vi "Matrix Inverse.vi"(2 "n":i32, 3 "A":sgl[](array[numeric])) -> (0 "divide by zero detected":bool, 1 "inv(A)":sgl[](array[numeric]))   [LabVIEW 2020]
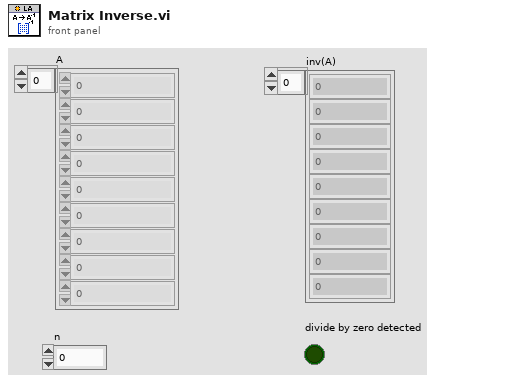
[diagram p1: front panel]
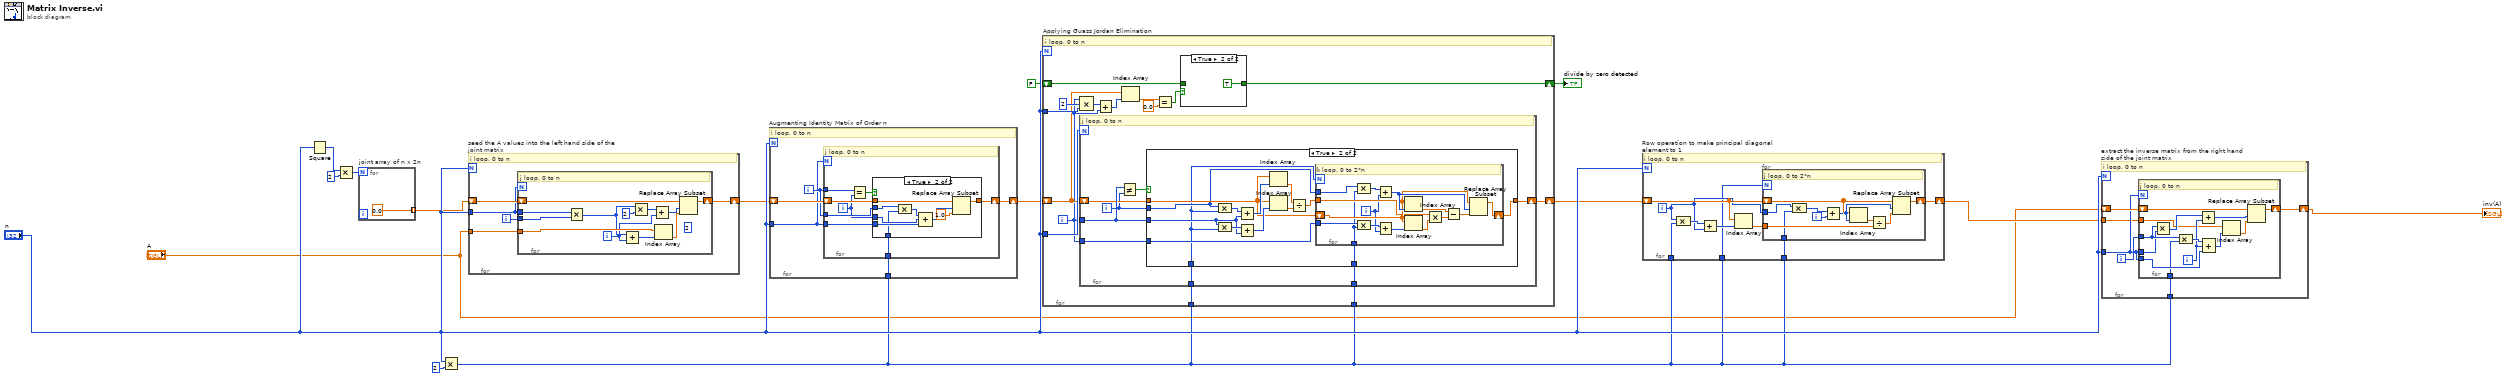
[diagram p0: block diagram]
diagram:
  n1 = Square(x="n") -> (x^2=w14:i32)
  n2 = Multiply(x=w14, y=2) -> (x*y=w2:i32)
  n3 = for "joint array of n x 2n" {
    N: w2 -> [_]
    tunnel: [sgl 0.0] -> w3 mode=indexing
  }
  n4 = Multiply(x="n", y=2) -> (x*y=w13:i32)
  n5 = for "seed the A values into the left hand side of the joint matrix" {
    N: "n" -> [_]
    shift-right: [w20] -> w4
    shift-left: w3 -> [w21]
    tunnel: "n" -> [w19]
    tunnel: "A" -> [w18]
    i -> [w17]
    # "i loop, 0 to n"
    n6 = for {
      N: w19 -> [_]
      shift-right: [w32] -> w20
      shift-left: w21 -> [w33]
      tunnel: w19 -> [w29]
      tunnel: w18 -> [w31]
      tunnel: w17 -> [w30]
      i -> [w23]
      (unwired) 2
      # "j loop, 0 to n"
      n7 = Multiply(x=w29, y=w30) -> (x*y=w25:i32)
      n8 = Add(x=w25, y=w23) -> (x+y=w28:i32)
      n9 = Multiply(x=w25, y=2) -> (x*y=w24:i32)
      n10 = Add(x=w24, y=w23) -> (x+y=w22:i32)
      n11 = Index Array(array=w31, index=w28) -> (element=w27:sgl)
      n12 = Replace Array Subset(array=w33, new element=w27, index=w22) -> (w32:sgl[])
    }
  }
  n13 = for "Augmenting Identity Matrix of Order n" {
    N: "n" -> [_]
    shift-right: [w37] -> w7
    shift-left: w4 -> [w38]
    tunnel: "n" -> [w35]
    tunnel: w13 -> [w34]
    i -> [w36]
    # "i loop, 0 to n"
    n14 = for {
      N: w35 -> [_]
      tunnel: w36 -> [w46]
      shift-right: [w43] -> w37
      shift-left: w38 -> [w44]
      tunnel: w36 -> [w42]
      tunnel: w35 -> [w41]
      tunnel: w34 -> [w39]
      i -> [w40]
      # "j loop, 0 to n"
      n15 = Equal?(x=w46, y=w40) -> (x = y?=w45:bool)
      n16 = case shown="True" w45 {
        tunnel: w44 -> [w47 w56]
        tunnel: [w47 w53] -> w43
        tunnel: w42 -> [_ w54]
        tunnel: w41 -> [_ w50]
        tunnel: w40 -> [_ w51]
        tunnel: w39 -> [_ w48]
        frame False {
        }
        frame True {
          n17 = Compound Arithmetic op=MULTIPLY(w54, w48) -> (w52:i32)
          n18 = Compound Arithmetic op=ADD(w52, w51, w50) -> (w49:i32)
          n19 = Replace Array Subset(array=w56, new element=sgl 1.0 ("new element/subarray"), index=w49) -> (w53:sgl[])
        }
      }
    }
  }
  n20 = for "Applying Guass Jordan Elimination" {
    N: "n" -> [_]
    tunnel: "n" -> [w69]
    shift-right: [w63] -> w6
    shift-left: FALSE -> [w64]
    tunnel: "n" -> [w62]
    shift-right: [w59] -> w8
    shift-left: w7 -> [w61]
    tunnel: w13 -> [w58]
    tunnel: w13 -> [w57]
    i -> [w60]
    # "i loop, 0 to n"
    n21 = Compound Arithmetic op=MULTIPLY(w60, 2 ("value"), w69) -> (w68:i32)
    n22 = for {
      N: w62 -> [_]
      tunnel: w60 -> [w79]
      tunnel: w60 -> [w75]
      shift-right: [w74] -> w59
      shift-left: w61 -> [w78]
      tunnel: w58 -> [w73]
      tunnel: w57 -> [w72]
      i -> [w76]
      # "j loop, 0 to n"
      n23 = Not Equal?(x=w79, y=w76) -> (x != y?=w77:bool)
      n24 = case shown="True" w77 {
        tunnel: w79 -> [_ w88]
        tunnel: w78 -> [w80 w87]
        tunnel: w76 -> [_ w86]
        tunnel: w75 -> [_ w84]
        tunnel: [w80 w83] -> w74
        tunnel: w73 -> [_ w82]
        tunnel: w72 -> [_ w81]
        frame False {
        }
        frame True {
          n25 = Compound Arithmetic op=MULTIPLY(w86, w82) -> (w94:i32)
          n26 = Compound Arithmetic op=MULTIPLY(w88, w82) -> (w90:i32)
          n27 = Add(x=w94, y=w88) -> (x+y=w93:i32)
          n28 = Add(x=w90, y=w88) -> (x+y=w89:i32)
          n29 = Index Array(array=w87, index=w93) -> (element=w92:sgl)
          n30 = Index Array(array=w87, index=w89) -> (element=w91:sgl)
          n31 = Divide(x=w92, y=w91) -> (x/y=w85:sgl)
          n32 = for {
            N: w82 -> [_]
            tunnel: w86 -> [w108]
            tunnel: w85 -> [w104]
            tunnel: w84 -> [w101]
            shift-right: [w96] -> w83
            shift-left: w87 -> [w106]
            tunnel: w81 -> [w95]
            i -> [w102]
            # "k loop, 0 to 2*n"
            n33 = Compound Arithmetic op=MULTIPLY(w108, w95) -> (w109:i32)
            n34 = Compound Arithmetic op=MULTIPLY(w101, w95) -> (w103:i32)
            n35 = Add(x=w109, y=w102) -> (x+y=w107:i32)
            n36 = Add(x=w103, y=w102) -> (x+y=w100:i32)
            n37 = Index Array(array=w106, index=w107) -> (element=w98:sgl)
            n38 = Index Array(array=w106, index=w100) -> (element=w105:sgl)
            n39 = Multiply(x=w104, y=w105) -> (x*y=w99:sgl)
            n40 = Subtract(x=w98, y=w99) -> (x-y=w97:sgl)
            n41 = Replace Array Subset(array=w106, new element=w97, index=w107) -> (w96:sgl[])
          }
        }
      }
    }
    n42 = Add(x=w68, y=w60) -> (x+y=w67:i32)
    n43 = Index Array(array=w61, index=w67) -> (element=w66:sgl)
    n44 = Equal?(x=w66, y=sgl 0.0) -> (x = y?=w65:bool)
    n45 = case shown="True" w65 {
      tunnel: w64 -> [w110 _]
      tunnel: [w110 TRUE] -> w63
      frame False {
      }
      frame True {
      }
    }
  }
  "divide by zero detected" <- w6
  n46 = for "Row operation to make principal diagonal element to 1" {
    N: "n" -> [_]
    shift-right: [w115] -> w11
    shift-left: w8 -> [w118]
    tunnel: w13 -> [w114]
    tunnel: w13 -> [w113]
    tunnel: w13 -> [w112]
    i -> [w117]
    # "i loop, 0 to n"
    n47 = Compound Arithmetic op=MULTIPLY(w117, w113) -> (w120:i32)
    n48 = Add(x=w120, y=w117) -> (x+y=w119:i32)
    n49 = Index Array(array=w118, index=w119) -> (element=w116:sgl)
    n50 = for {
      N: w114 -> [_]
      tunnel: w117 -> [w130]
      tunnel: w116 -> [w126]
      shift-right: [w124] -> w115
      shift-left: w118 -> [w125]
      tunnel: w112 -> [w121]
      i -> [w128]
      # "j loop, 0 to 2*n"
      n51 = Compound Arithmetic op=MULTIPLY(w130, w121) -> (w129:i32)
      n52 = Add(x=w129, y=w128) -> (x+y=w123:i32)
      n53 = Index Array(array=w125, index=w123) -> (element=w127:sgl)
      n54 = Divide(x=w127, y=w126) -> (x/y=w122:sgl)
      n55 = Replace Array Subset(array=w125, new element=w122, index=w123) -> (w124:sgl[])
    }
  }
  n56 = for "extract the inverse matrix from the right hand side of the joint matrix" {
    N: "n" -> [_]
    tunnel: "n" -> [w133]
    shift-right: [w135] -> w10
    shift-left: "A" -> [w136]
    tunnel: w11 -> [w132]
    tunnel: w13 -> [w131]
    i -> [w134]
    # "i loop, 0 to n"
    n57 = for {
      N: w133 -> [_]
      shift-right: [w148] -> w135
      shift-left: w136 -> [w149]
      tunnel: w134 -> [w145]
      tunnel: w133 -> [w144]
      tunnel: w133 -> [w141]
      tunnel: w132 -> [w139]
      tunnel: w131 -> [w137]
      i -> [w142]
      # "j loop, 0 to n"
      n58 = Multiply(x=w145, y=w144) -> (x*y=w147:i32)
      n59 = Compound Arithmetic op=MULTIPLY(w145, w137) -> (w143:i32)
      n60 = Add(x=w147, y=w142) -> (x+y=w146:i32)
      n61 = Compound Arithmetic op=ADD(w143, w142, w141) -> (w140:i32)
      n62 = Index Array(array=w139, index=w140) -> (element=w138:sgl)
      n63 = Replace Array Subset(array=w149, new element=w138, index=w146) -> (w148:sgl[])
    }
  }
  "inv(A)" <- w10
